vi "Config_LoadCreate.vi"(7 "Config In":path, 8 "error In":errorcluster, 10 "Configuration Cluster":T1={"General"={"Config.ini"=path "", "Default Logging Path"=path ""}, "Hardware"={"AHC VISA COM"="", "Measure Rate (1/s)"=0, "Global T VAR"="", "Global B VAR"=""}, "Operation"={"Operation Mode"=enum."Idle-Off", "Status"="", "NewLog?"=FALSE}}, 11 "AH VISA COM":refnum<visa-resource-name>) -> (0 "error out":errorcluster, 2 "Configuration Cluster Out":T1={"General"={"Config.ini"=path "", "Default Logging Path"=path ""}, "Hardware"={"AHC VISA COM"="", "Measure Rate (1/s)"=0, "Global T VAR"="", "Global B VAR"=""}, "Operation"={"Operation Mode"=enum."Idle-Off", "Status"="", "NewLog?"=FALSE}}, 3 "AHC VISA COM Out":refnum<visa-resource-name>)   [LabVIEW 2021]
uses:
  Config_Cluster.ctl
  Mode_Enum.ctl
  <vilib>/Utility/config.llb/Read Key (Path).vi
  <vilib>/Utility/config.llb/NI_LVConfig.lvlib
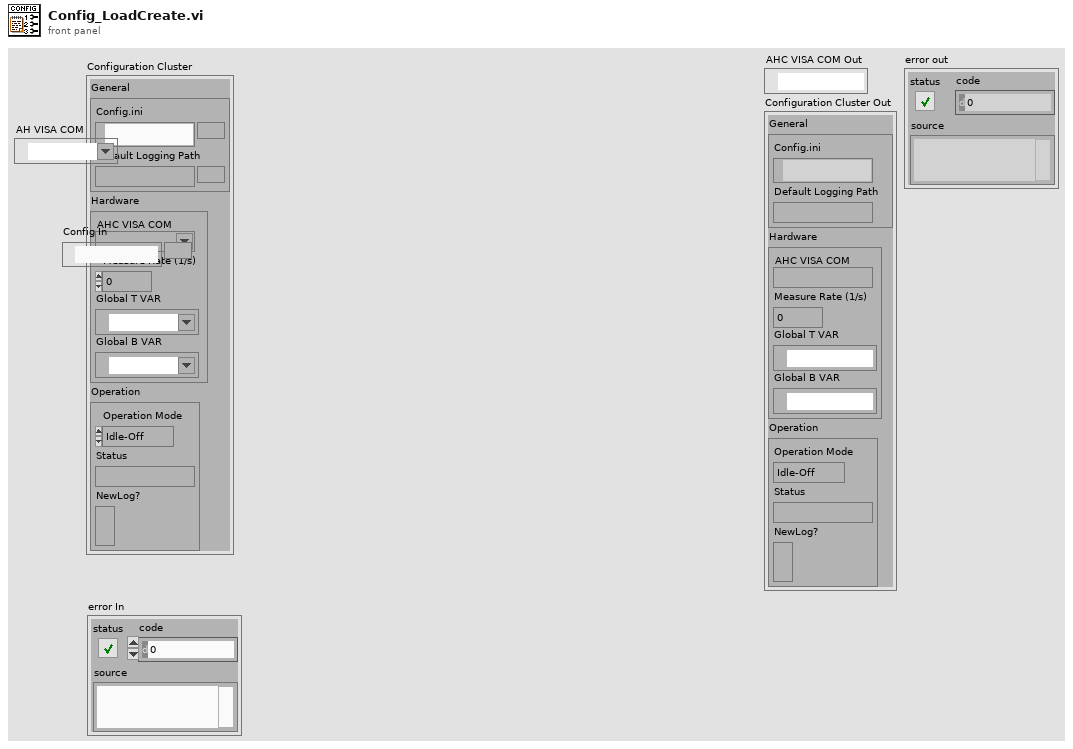
[diagram p1: front panel]
types:
  T1 = typedef "Config_Cluster.ctl" = cluster{"General":cluster{"Config.ini":path, "Default Logging Path":path}, "Hardware":cluster{"AHC VISA COM":refnum<visa-resource-name>, "Measure Rate (1/s)":i32, "Global T VAR":refnum<k21>, "Global B VAR":refnum<k21>}, "Operation":cluster{"Operation Mode":T2, "Status":string, "NewLog?":bool}}
  T2 = typedef "Mode_Enum.ctl" = enum16{"Logging", "Idle-Off", "Idle"}
  T3 = typedef "NI_LVConfig.lvlib/Config Data RefNum.ctl" = refnum<k1>
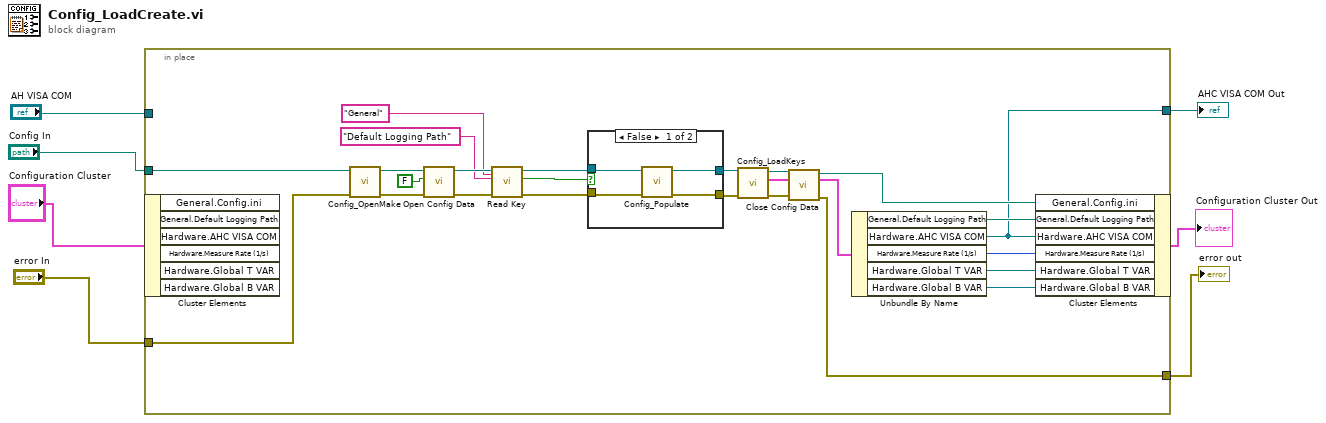
[diagram p0: block diagram]
diagram:
  n1 = in-place {
    in-place-border: "AH VISA COM" -> [_]
    in-place-border: "error In" -> [w30]
    in-place-border: "Config In" -> [w31]
    in-place-border: [w11] -> w3
    in-place-border: [w10] -> w1
    n2 = in-place-cluster #1("Configuration Cluster") -> ()  [unwired: 6 out]
    n3 = call "Config_OpenMake.vi"("error in (no error)"=w30, "Config Path"=w31) -> ("error out"=w27:errorcluster, "File Path"=w29:path)  [unwired: 8 in]
    n4 = call <vilib>:"Open Config Data.vi"("error in (no error)"=w27, "create file if necessary (T)"=FALSE, "configuration file path"=w29) -> ("error out"=w25:errorcluster, "refnum"=w26:T3)  [unwired: 6 in, 1 out]
    n5 = call-poly <vilib>:"Read Key.vi"("section"="General", "error in (no error)"=w25, "key"="Default Logging Path", "refnum"=w26) -> ("error out"=w21:errorcluster, "found?"=w20:bool, "refnum out"=w22:T3)  [unwired: 4 in, 1 out]
    n6 = case shown="False" w20 {
      tunnel: w21 -> [w34 w36]
      tunnel: w22 -> [w35 w37]
      tunnel: [w33 w36] -> w16
      tunnel: [w32 w37] -> w18
      frame False {
        n7 = call "Config_Populate.vi"("error in (no error)"=w34, "Config Ref In"=w35) -> ("error out"=w33:errorcluster, "refnum out"=w32:T3)  [unwired: 8 in]
      }
      frame True {
      }
    }
    n8 = call "Config_LoadKeys.vi"("error in (no error)"=w16, "Config In"=w18) -> ("error out"=w15:errorcluster, "output cluster"=w14:T1, "refnum out"=w17:T3)  [unwired: 7 in]
    n9 = call <vilib>:"Close Config Data.vi"("error in (no error)"=w15, "refnum"=w17) -> ("error out"=w10:errorcluster, "file path"=w19:path)  [unwired: 8 in]
    n10 = Unbundle By Name(w14) -> ("General.Default Logging Path"=w13:path, "Hardware.AHC VISA COM"=w11:refnum<visa-resource-name>, "Hardware.Measure Rate (1/s)"=w12:i32, "Hardware.Global T VAR"=w9:refnum<k21>, "Hardware.Global B VAR"=w8:refnum<k21>)
    n11 = in-place-cluster #1("General.Config.ini"=w19, "General.Default Logging Path"=w13, "Hardware.AHC VISA COM"=w11, "Hardware.Measure Rate (1/s)"=w12, "Hardware.Global T VAR"=w9, "Hardware.Global B VAR"=w8) -> (→"Configuration Cluster Out":T1)
  }
  "AHC VISA COM Out" <- w3
  "error out" <- w1
